vi "Inspect.vi"(9 "Msg":refnum<class "Msg.lvclass">, 10 "Within Msg Set":bool, 11 "Actor in":refnum<class "Actor.lvclass">) -> (2 "Proceed":bool=TRUE, 3 "Actor out":refnum<class "Actor.lvclass">)   [LabVIEW 2025, in "jettl.lvlib" / "Actor.lvclass"]
uses:
  Actor.lvclass
  Msg/Msg.lvclass
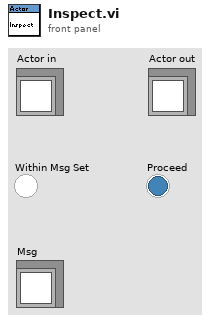
[diagram p1: front panel]
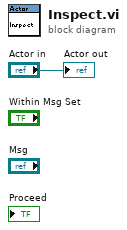
[diagram p0: block diagram]
diagram:
  "Actor out" <- "Actor in"
